vi "ALARM Update.vi"(8 "error in (no error)":errorcluster, 10 "Message Data":variant, 11 "Data Cluster":T1={"LOG REF"=refnum, "Writer Queue"=refnum, "Log Path"=path "", "UPS standby"=FALSE, "status code"=5001, "SP"=[], "Over Sens Status"=[]}) -> (0 "error out":errorcluster, 3 "Data Cluster out":T1={"LOG REF"=refnum, "Writer Queue"=refnum, "Log Path"=path "", "UPS standby"=FALSE, "status code"=5001, "SP"=[], "Over Sens Status"=[]})   [LabVIEW 2020, in "QCT ALARM.lvlib"]
uses:
  QCT ALARM.lvlib
  ALARM Configuration.ctl
  support/Message Queue/Message Cluster.ctl
  support/Message Queue/Message Queue.lvlib
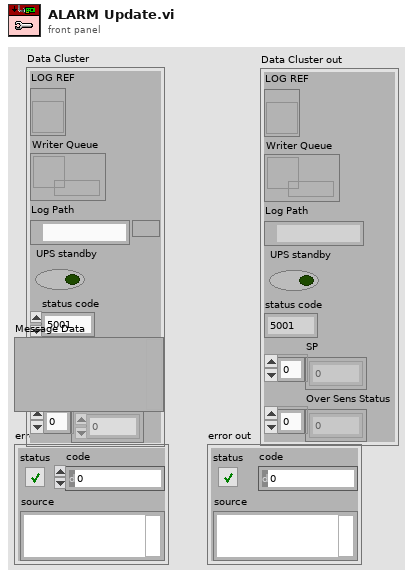
[diagram p1: front panel]
types:
  T1 = typedef "QCT ALARM.lvlib/ALARM Configuration.ctl" = cluster{"LOG REF":refnum<vi>, "Writer Queue":refnum<queue>, "Log Path":path, "UPS standby":bool, "status code":i32, "SP":dbl[], "Over Sens Status":dbl[]}
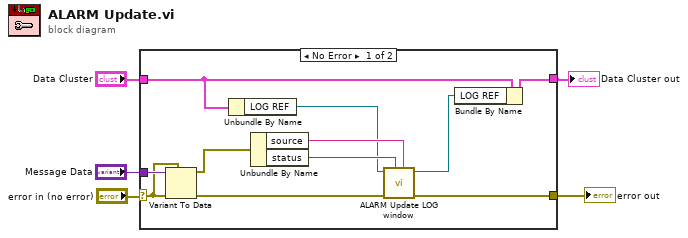
[diagram p0: block diagram]
diagram:
  n1 = case shown="No Error" "error in (no error)" {
    selector: "error in (no error)" -> [w12 w17]
    tunnel: [w7 w18] -> w4
    tunnel: "Data Cluster" -> [w9 w18]
    tunnel: [w14 w17] -> w3
    tunnel: "Message Data" -> [w13 _]
    frame No Error {
      n2 = Variant To Data(error in=w12, type=w12, Variant=w13) -> (data=w16:errorcluster, error out=w15:errorcluster)
      n3 = Unbundle By Name(w9) -> ("LOG REF"=w8:refnum<vi>)
      n4 = Unbundle By Name(w16) -> ("source"=w11:string, "status"=w10:bool)
      n5 = call "ALARM Update LOG window.vi"("String"=w11, "replace"=w10, "error in (no error)"=w15, "strLOG in"=w8) -> ("error out"=w14:errorcluster, "strLOG out"=w6:refnum<vi>)  [unwired: 6 in]
      n6 = Bundle By Name(cluster=w9, "LOG REF"=w6) -> (w7:T1)
    }
    frame Error {
    }
  }
  "error out" <- w3
  "Data Cluster out" <- w4
